vi "Read.vi"(6 "Timeout (1000 ms)":u16=1000, 8 "error in (no error)":errorcluster, 9 "Bytes to Read":u8, 10 "I2C Slave Address":u8, 11 "I2C Linx in":refnum<class "LinxI2C.lvclass">) -> (0 "error out":errorcluster, 2 "Data":u8[](array[numeric]), 3 "I2C Linx out":refnum<class "LinxI2C.lvclass">)   [LabVIEW 2014, in "LinxI2C.lvclass"]
doc: "Read the specified number of bytes from the I2C slave at the specified address."
uses:
  LinxI2C.lvclass
  LinxI2C.lvclass/LinxI2C.ctl
  <vilib>/MakerHub/LINX/LMH-LINX.lvlib
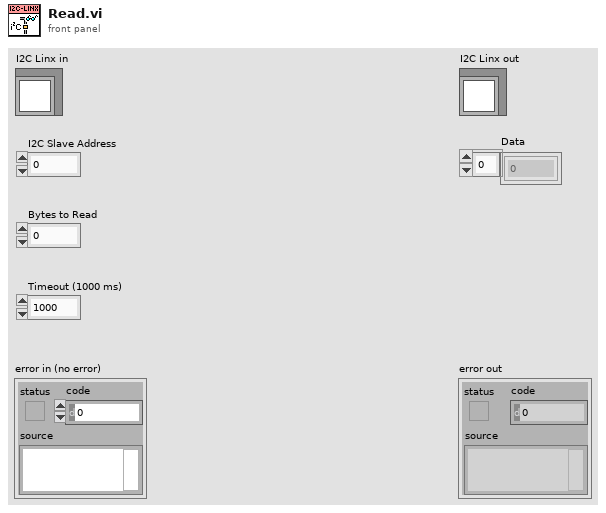
[diagram p1: front panel]
types:
  T1 = typedef "LMH-LINX.lvlib/LINX Ref.ctl" = cluster{"IO":T2, "Interface":T3, "LINX Device Config":T4}
  T2 = typedef "LMH-LINX.lvlib/Platform.ctl" = enum16{"Remote", "Local"}
  T3 = typedef "LMH-LINX.lvlib/Interface.ctl" = enum16{"Serial", "TCP"}
  T4 = typedef "LMH-LINX.lvlib/Device.lvlib/LINX Device Config.ctl" = cluster{"Interface":T3, "COM Port":refnum<visa-resource-name>, "TCP Configuration":T5, "Device Family":u8, "Device ID":u8, "Device Name":string, "TCP Ref":refnum<k5>, "Channels":T6}
  T5 = typedef "LMH-LINX.lvlib/Device.lvlib/TCP Config.ctl" = cluster{"IP Address":string, "Port":u16}
  T6 = typedef "LMH-LINX.lvlib/Channels.ctl" = cluster{"DI":u8[], "DO":u8[], "AI":u8[], "AO":u8[], "PWM":u8[], "QE":u8[], "UART":u8[], "I2C 2":u8[], "SPI":u8[], "CAN":u8[], "Servo":u8[], "AI Ref (V)":dbl, "AI Resolution (Bits)":u8, "AO Ref (V)":dbl, "AO Resolution (Bits)":u8}
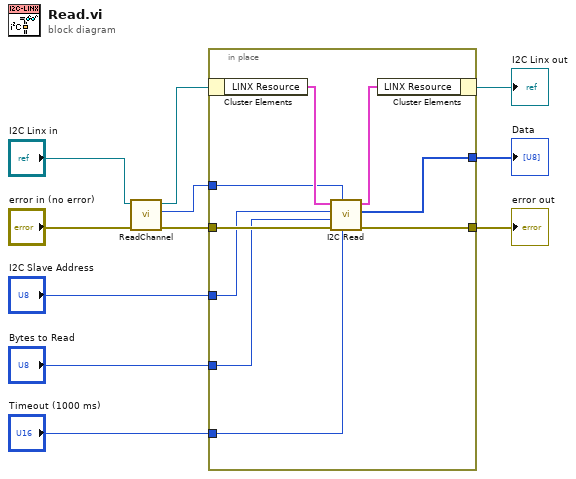
[diagram p0: block diagram]
diagram:
  n1 = call-dynamic "ReadChannel.vi"("error in (no error)"="error in (no error)", "I2C in"="I2C Linx in") -> ("error out"=w11:errorcluster, "I2C Channel"=w9:u8, "I2C out"=w10:refnum<class "LinxI2C.lvclass">)  [unwired: 7 in]
  n2 = in-place {
    in-place-border: w11 -> [w20]
    in-place-border: [w16] -> w3
    in-place-border: w9 -> [w17]
    in-place-border: "I2C Slave Address" -> [w15]
    in-place-border: "Bytes to Read" -> [w14]
    in-place-border: "Timeout (1000 ms)" -> [w13]
    in-place-border: [w12] -> w2
    n3 = in-place-cluster #1(w10) -> ("LINX Resource"=w19:T1)
    n4 = call <vilib>:"I2C Read.vi"("Timeout (1000 ms)"=w13, "I2C Channel"=w17, "Error In"=w20, "Bytes To Read"=w14, "I2C Slave Address (0)"=w15, "LINX Resource"=w19) -> ("Error Out"=w16:errorcluster, "Data"=w12:u8[], "LINX Resource"=w18:T1)  [unwired: 3 in]
    n5 = in-place-cluster #1("LINX Resource"=w18) -> (→"I2C Linx out":refnum<class "LinxI2C.lvclass">)
  }
  "error out" <- w3
  "Data" <- w2
